vi "get Pmu Configuration Ver3.vi"(9 "pmuIndex":i32, 10 "pseudoPdcId":i32, 11 "pmuconf":T1) -> (1 "function return":i32, 2 "stationname":string, 3 "pmuconf out":T1)   [LabVIEW 2013, in "C37118-DLL.lvlib" / "StrongridDLL.lvlib"]
doc: "STRONGRIDIEEEC37118DLL_API int __cdecl getPmuConfiguration_Ver3(pmuConfig_Ver3* pmuconf, int32_t pseudoPdcId, int32_t pmuIndex);"
uses:
  StrongridDLL.lvlib
  <vilib>/Utility/importsl/GetValueByPointer/datatype.ctl
  <vilib>/Utility/importsl/GetValueByPointer/GetValueByPointer.xnode
  <vilib>/S3DK/data/StrongridDLL.dll
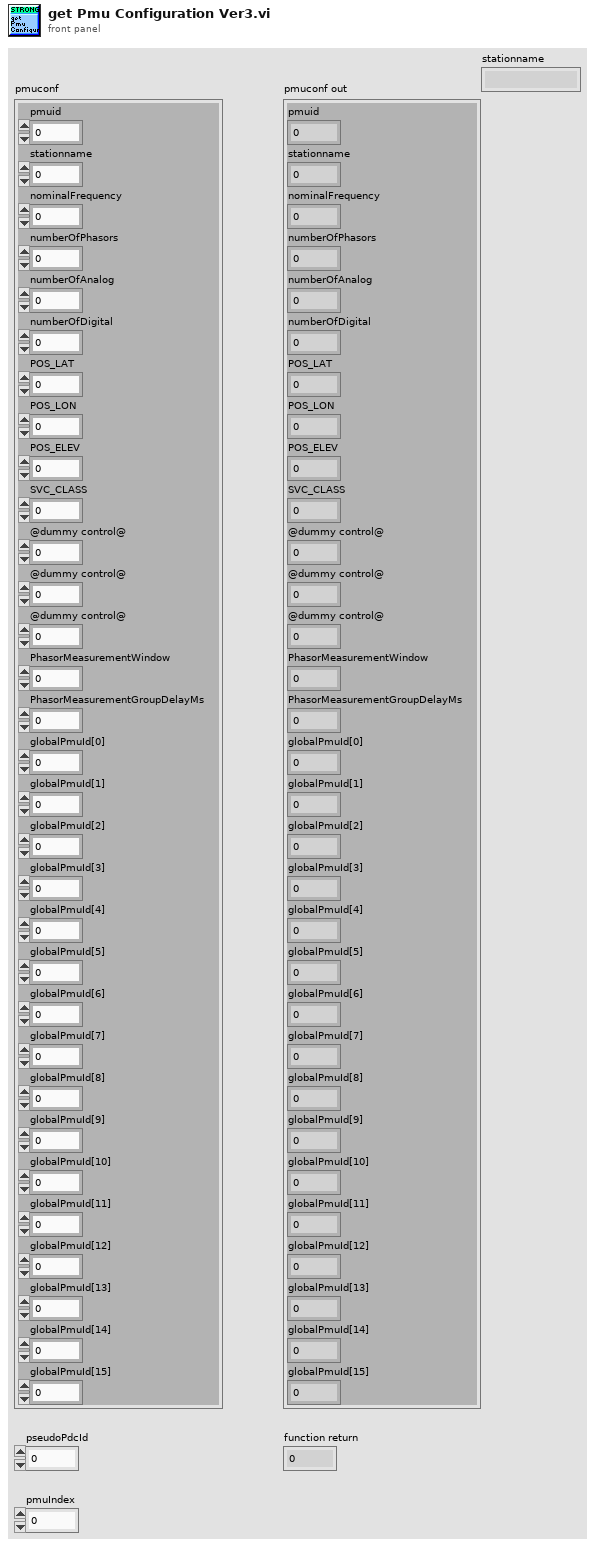
[diagram p1: front panel]
types:
  T1 = cluster{"pmuid":i32, "stationname":u32, "nominalFrequency":sgl, "numberOfPhasors":i32, "numberOfAnalog":i32, "numberOfDigital":i32, "POS_LAT":sgl, "POS_LON":sgl, "POS_ELEV":sgl, "SVC_CLASS":u8, "@dummy control@":i8, "@dummy control@":i8, "@dummy control@":i8, "PhasorMeasurementWindow":i32, "PhasorMeasurementGroupDelayMs":i32, "globalPmuId[0]":i8, "globalPmuId[1]":i8, "globalPmuId[2]":i8, "globalPmuId[3]":i8, "globalPmuId[4]":i8, "globalPmuId[5]":i8, "globalPmuId[6]":i8, "globalPmuId[7]":i8, "globalPmuId[8]":i8, "globalPmuId[9]":i8, "globalPmuId[10]":i8, "globalPmuId[11]":i8, "globalPmuId[12]":i8, "globalPmuId[13]":i8, "globalPmuId[14]":i8, "globalPmuId[15]":i8}
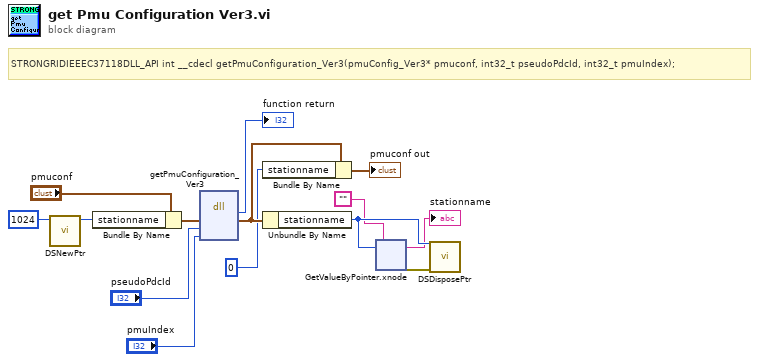
[diagram p0: block diagram]
diagram:
  # "STRONGRIDIEEEC37118DLL_API int __cdecl getPmuConfiguration_Ver3(pmuConfig_Ver3* pmuconf, int32_t pseudoPdcId, int32_t pmuIndex);"
  n1 = call <vilib>:"DSNewPtr.vi"("Size"=u64 1024) -> ("Pointer"=w11:u64)  [unwired: 9 in, 1 out]
  n2 = Bundle By Name(cluster="pmuconf", "stationname"=w11) -> (w10:T1)
  n3 = dll-call lib="C:/Program Files (x86)/National Instruments/LabVIEW 2013/vi.lib/S3DK/data/StrongridDLL.*" fn="getPmuConfiguration_Ver3"("pmuconf"=w10, "pseudoPdcId"="pseudoPdcId", "pmuIndex"="pmuIndex") -> (→"function return":i32, "pmuconf"=w5:T1)  [unwired: 5 in, 2 out]
  n4 = Bundle By Name(cluster=w5, "stationname"=u32 0) -> (→"pmuconf out":T1)
  n5 = Unbundle By Name(w5) -> ("stationname"=w8:u32)
  n6 = xnode "GetValueByPointer.xnode"("Pointer"=w8, "InputType"="") -> ("Output"=→"stationname":string, "ErrorOut"=w9:errorcluster)  [unwired: 2 in]
  n7 = call <vilib>:"DSDisposePtr.vi"("error in (no error)"=w9, "Pointer"=w8) -> ()  [unwired: 9 in, 1 out]
